vi "9219_AdjustUILayout.vi"(11 "Channels Refnum":refnum<vi>) -> ()   [LabVIEW 2017, in "Modules.lvlib" / "9219.lvclass"]
uses:
  9219.lvclass
  <vilib>/Utility/miscctls.llb/LVRowAndColumnTypeDef.ctl
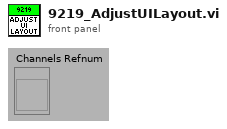
[diagram p1: front panel]
types:
  T1 = typedef "LVRowAndColumnTypeDef.ctl" = cluster{"Row":i32, "Column":i32}
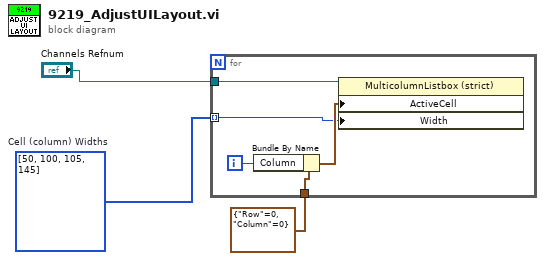
[diagram p0: block diagram]
diagram:
  w1 = u32[] [50, 100, 105, 145]  # Cell (column) Widths
  n1 = for {
    tunnel: "Channels Refnum" -> [w8]
    tunnel: T1 {"Row"=0, "Column"=0} ("Active Cell:Active Cell") -> [w7]
    tunnel: w1 -> [w4] mode=indexing
    i -> [w6]
    n2 = Bundle By Name(cluster=w7, "Column"=w6) -> (w5:T1)
    n3 = property class="MulticolumnListbox (strict)"(reference=w8, "ActiveCell"=w5, "Width"=w4) -> ()  [unwired: 1 in, 2 out]
  }
